vi "NI9234_SUB-VI_Queue.vi"(6 "Method":T1, 8 "error in (no error)":errorcluster, 11 "Cluster_SaveData":T2) -> (0 "error out":errorcluster, 2 "elements":T2[](array[typedef]), 3 "queue out":refnum<queue>)   [LabVIEW 2020]
uses:
  RPA_BACKDRIVE/GUI/SUBVI/TYPEDEF/ClusterSaveData.ctl
  RPA_BACKDRIVE/GUI/SUBVI/TYPEDEF/SaveData.ctl
  TYPEDEF/NI9234_TD_Method_Queue.ctl
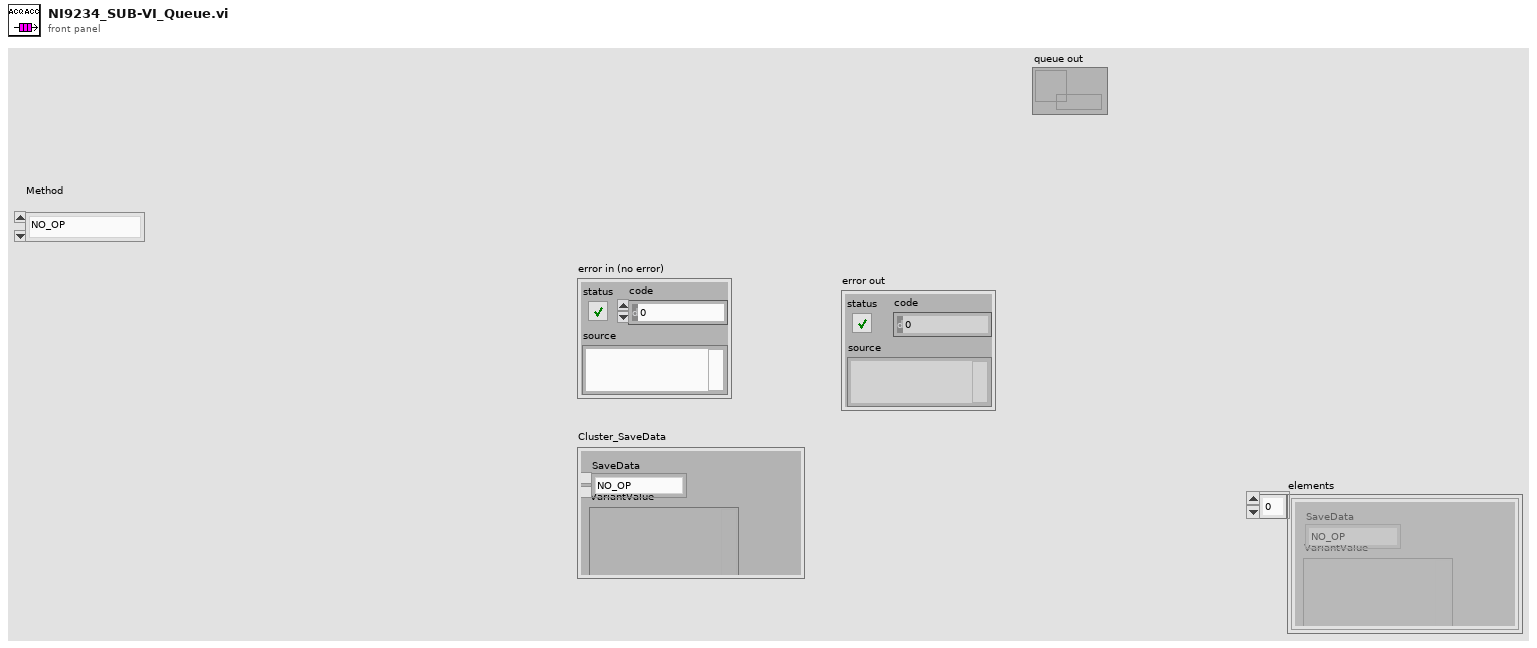
[diagram p1: front panel]
types:
  T1 = typedef "NI9234_TD_Method_Queue.ctl" = enum16{"NO_OP", "CREATE", "POPULATE", "FLUSH", "DESTROY", "DEL_ELEM", "GET_STATUS"}
  T2 = typedef "ClusterSaveData.ctl" = cluster{"VariantValue":variant, "SaveData":T3}
  T3 = typedef "SaveData.ctl" = enum16{"NO_OP", "FUNZIONE", "INVIA_DATI", "RILETTURA"}
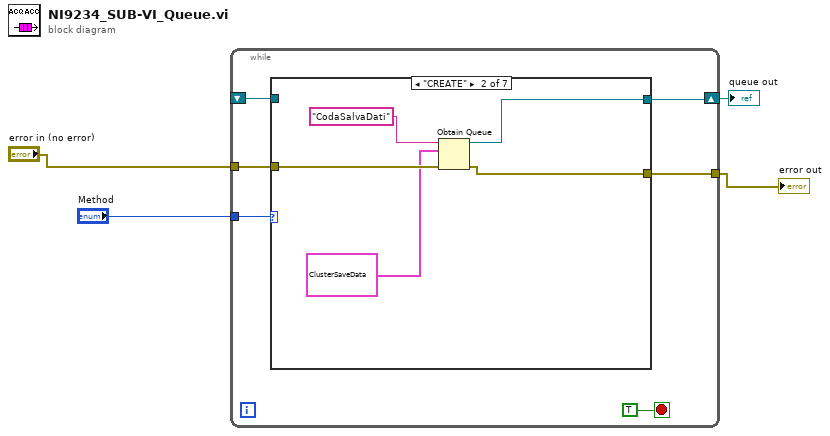
[diagram p0: block diagram]
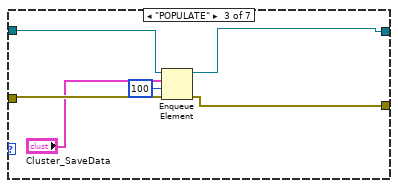
[diagram p3: hidden frame]
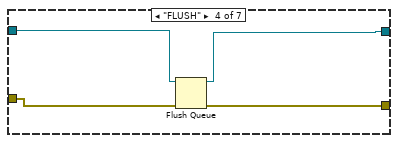
[diagram p4: hidden frame]
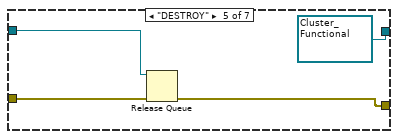
[diagram p5: hidden frame]
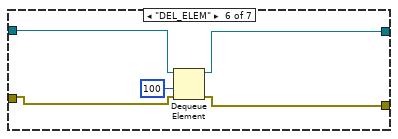
[diagram p6: hidden frame]
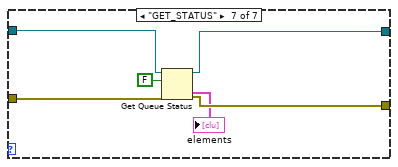
[diagram p7: hidden frame]
diagram:
  n1 = while {
    tunnel: "Method" -> [w10]
    tunnel: [w9] -> w2
    tunnel: "error in (no error)" -> [w8]
    shift-right: [w6] -> w1
    shift-left: _ -> [w5]
    stop <- TRUE stop-if-true
    n2 = case shown="\"CREATE\"" w10 {
      tunnel: [w12 w16 w21 w26 w31 w33 w40] -> w9
      tunnel: w8 -> [w12 w17 w20 w27 w30 w34 w38]
      tunnel: [w11 w14 w22 w24 refnum<queue> refnum ("queue out") w32 w41] -> w6
      tunnel: w5 -> [w11 _ w23 w25 w29 w36 w42]
      frame "NO_OP" {
      }
      frame "CREATE" {
        n3 = Obtain Queue(name (unnamed)="CodaSalvaDati", element data type=T2 {"VariantValue"=variant, "SaveData"=enum."NO_OP"} ("Cluster_Functional"), error in (no error)=w17) -> (queue out=w14:refnum<queue>, error out=w16:errorcluster)  [unwired: 2 in, 1 out]
      }
      frame "POPULATE" {
        n4 = Enqueue Element(queue=w23, element="Cluster_SaveData", timeout in ms (-1)=100, error in (no error)=w20) -> (queue out=w22:refnum<queue>, error out=w21:errorcluster)  [unwired: 1 out]
      }
      frame "FLUSH" {
        n5 = Flush Queue(queue=w25, error in (no error)=w27) -> (queue out=w24:refnum<queue>, error out=w26:errorcluster)  [unwired: 1 out]
      }
      frame "DESTROY" {
        n6 = Release Queue(queue=w29, error in (no error)=w30) -> (error out=w31:errorcluster)  [unwired: 1 in, 2 out]
      }
      frame "DEL_ELEM" {
        n7 = Dequeue Element(queue=w36, timeout in ms (-1)=100, error in (no error)=w34) -> (queue out=w32:refnum<queue>, error out=w33:errorcluster)  [unwired: 2 out]
      }
      frame "GET_STATUS" {
        n8 = Get Queue Status(queue=w42, return elements? (F)=FALSE, error in (no error)=w38) -> (queue out=w41:refnum<queue>, error out=w40:errorcluster, elements=→"elements":T2[])  [unwired: 5 out]
      }
    }
  }
  "error out" <- w2
  "queue out" <- w1
